vi "Rename Class Controls.vi"(6 "Old Class":path, 8 "error in":errorcluster, 9 "Class to Rename":refnum<vi>, 10 "App Ref":refnum<vi>) -> (0 "error out":errorcluster)   [LabVIEW 2021, in "_Rename.lvlib" / "SAS.lvlib"]
uses:
  <vilib>/Utility/traverseref.llb/TRef TravTarget.ctl
  SAS.lvlib
  <vilib>/Utility/traverseref.llb/VI Scripting - Traverse.lvlib
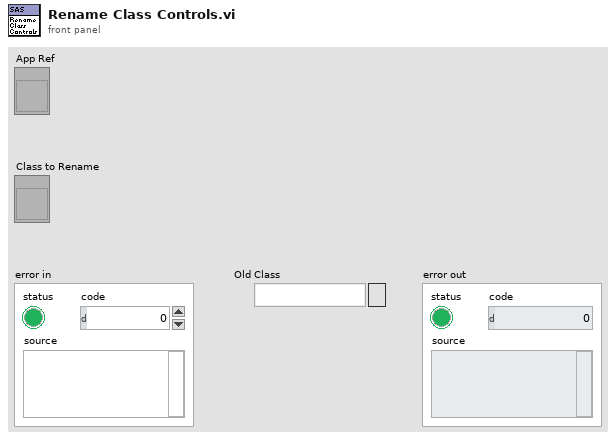
[diagram p1: front panel]
types:
  T1 = typedef "TRef TravTarget.ctl" = enum16{"FP", "BD", "Other"}
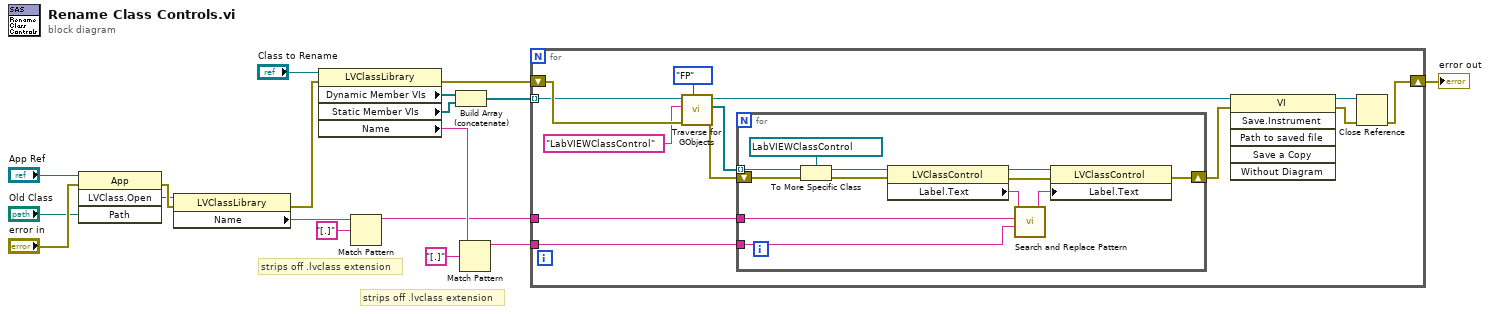
[diagram p0: block diagram]
diagram:
  # "strips off .lvclass extension"
  # "strips off .lvclass extension"
  n1 = invoke class="App" method="LVClass.Open"(reference="App Ref", error in="error in", "Path"="Old Class") -> (error out=w17:errorcluster, "LVClass.Open"=w12:refnum<vi>)  [unwired: 1 in, 2 out]
  n2 = property class="LVClassLibrary"(reference=w12, error in=w17) -> (error out=w18:errorcluster, "Name"=w11:string)  [unwired: 1 out]
  n3 = property class="LVClassLibrary"(reference="Class to Rename", error in=w18) -> (error out=w15:errorcluster, "Dynamic Member VIs"=w3:refnum<vi>[], "Static Member VIs"=w4:refnum<vi>[], "Name"=w9:string)  [unwired: 1 out]
  n4 = Match Pattern(string=w11, regular expression="[.]") -> (before substring=w2:string)  [unwired: 1 in, 3 out]
  n5 = Build Array (concatenate)(w3, w4) -> (w5:refnum<vi>[])
  n6 = Match Pattern(string=w9, regular expression="[.]") -> (before substring=w8:string)  [unwired: 1 in, 3 out]
  n7 = for {
    tunnel: w5 -> [w26] mode=indexing
    tunnel: w8 -> [w19]
    tunnel: w2 -> [w22]
    shift-right: [w27] -> w14
    shift-left: w15 -> [w31]
    n8 = call <vilib>:"Traverse for GObjects.vi"("Traverse Target"=TRef_TravTarget."FP", "error in (no error)"=w31, "Class Name"="LabVIEWClassControl", "VI Refnum"=w26) -> ("error out"=w30:errorcluster, "References"=w23:refnum<vi>[], "dup VI Refnum"=w20:refnum<vi>)  [unwired: 4 in, 1 out]
    n9 = for {
      tunnel: w23 -> [w39] mode=indexing
      tunnel: w19 -> [w35]
      tunnel: w22 -> [w33]
      shift-right: [w40] -> w29
      shift-left: w30 -> [w41]
      n10 = To More Specific Class(target class=refnum<vi> refnum ("LVClassControl Refnum"), reference=w39, error in=w41) -> (specific class reference=w38:refnum<vi>, error out=w43:errorcluster)
      n11 = property class="LVClassControl"(reference=w38, error in=w43) -> (reference out=w37:refnum<vi>, error out=w42:errorcluster, "Label.Text"=w36:string)
      n12 = call <vilib>:"Search and Replace Pattern.vi"("string"=w36, "regular expression (\"\")"=w33, "replace string (\"\")"=w35) -> ("result string"=w34:string)  [unwired: 2 in, 1 out]
      n13 = property class="LVClassControl"(reference=w37, error in=w42, "Label.Text"=w34) -> (error out=w40:errorcluster)  [unwired: 1 out]
    }
    n14 = invoke class="VI" method="Save.Instrument"(reference=w20, error in=w29) -> (reference out=w21:refnum<vi>, error out=w28:errorcluster)  [unwired: 4 in, 4 out]
    n15 = Close Reference(reference=w21, error in (no error)=w28) -> (error out=w27:errorcluster)
  }
  "error out" <- w14
